vi "PathPlanner_FileUtil_AddExt.vi"(9 "Extension":string="txt", 11 "Path in":path) -> (3 "Path out":path)   [LabVIEW 2019, in "PathPlanner24.lvlib"]
uses:
  PathPlanner24.lvlib
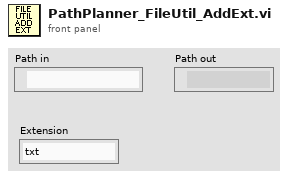
[diagram p1: front panel]
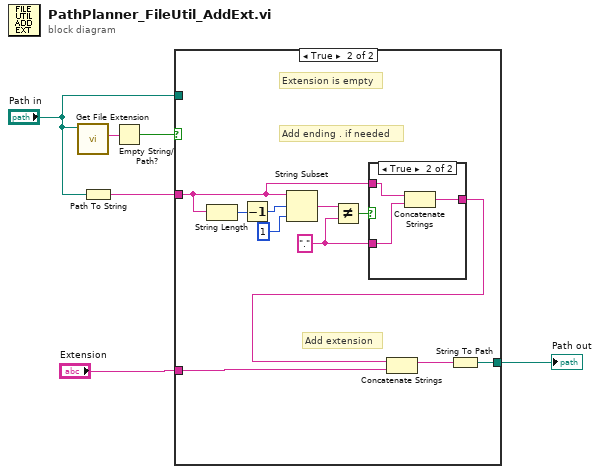
[diagram p0: block diagram]
diagram:
  n1 = call <vilib>:"Get File Extension.vi"("file"="Path in") -> ("lowercase file extension"=w4:string)  [unwired: 6 in, 4 out]
  n2 = Path To String(path="Path in") -> (string=w6:string)
  n3 = Empty String/Path?(string/path=w4) -> (empty?=w2:bool)
  n4 = case shown="True" w2 {
    tunnel: "Path in" -> [w7 _]
    tunnel: [w7 w10] -> w3
    tunnel: w6 -> [_ w13]
    tunnel: "Extension" -> [_ w8]
    frame False {
    }
    frame True {
      w12 = "."
      # "Add extension"
      # "Add ending . if needed"
      # "Extension is empty"
      n5 = String Length(string=w13) -> (length=w18:i32)
      n6 = Decrement(x=w18) -> (x-1=w17:i32)
      n7 = String Subset(string=w13, offset (0)=w17, length (rest)=1 ("length (rest)")) -> (substring=w15:string)
      n8 = Not Equal?(x=w15, y=w12) -> (x != y?=w14:bool)
      n9 = case shown="True" w14 {
        tunnel: w13 -> [w19 w22]
        tunnel: w12 -> [_ w21]
        tunnel: [w19 w20] -> w11
        frame False {
        }
        frame True {
          n10 = Concatenate Strings(w22, w21) -> (w20:string)
        }
      }
      n11 = Concatenate Strings(w11, w8) -> (w9:string)
      n12 = String To Path(string=w9) -> (path=w10:path)
    }
  }
  "Path out" <- w3
